vi "V1.0 Convert.vi"(11 "Old":T17 {"AllCaliperEntries"."CaliperType" items=["Distance", "Mid Point", "Perpendicular Projection", "Lines Intersection", "Angle from Horizontal", "Angle from Vertical", "Angle Defined by 3 Points", "Angle Defined by 4 Points", "Bissecting Line", "Mid Line", "Center of Mass", "Area", "Line Fit", "Circle Fit", "Ellipse Fit"]; "CoordinatteEntry Output"."AnalysisSetting"."OriginPointInfo"."Mode" items=["Horizontal Motion", "Vertical Motion", "Horizontal and Vertical Motion", "Horizontal. Vertical and Angular Motion"]; "CoordinatteEntry Output"."AnalysisSetting"."ROI"."Contours"."Type" items=["No Selection", "Point", "Line", "Rectangle", "Oval", "Polygon", "Freehand Region", "Annulus", "Unused2", "Unused3", "Broken Line", "Freehand Line", "Rotated Rectangle"]; "AllCaliperEntries"."CaliperType" items=["Distance", "Mid Point", "Perpendicular Projection", "Lines Intersection", "Angle from Horizontal", "Angle from Vertical", "Angle Defined by 3 Points", "Angle Defined by 4 Points", "Bissecting Line", "Mid Line", "Center of Mass", "Area", "Line Fit", "Circle Fit", "Ellipse Fit"]}) -> (3 "NewOut":T16 {"AllCaliperEntries"."CaliperType" items=["Distance", "Mid Point", "Perpendicular Projection", "Lines Intersection", "Angle from Horizontal", "Angle from Vertical", "Angle Defined by 3 Points", "Angle Defined by 4 Points", "Bissecting Line", "Mid Line", "Center of Mass", "Area", "Line Fit", "Circle Fit", "Ellipse Fit"]; "CoordinatteEntry Output"."CaliperSetting"."CaliperEntry"."CaliperType" items=["Distance", "Mid Point", "Perpendicular Projection", "Lines Intersection", "Angle from Horizontal", "Angle from Vertical", "Angle Defined by 3 Points", "Angle Defined by 4 Points", "Bissecting Line", "Mid Line", "Center of Mass", "Area", "Line Fit", "Circle Fit", "Ellipse Fit"]; "CoordinatteEntry Output"."OriginPointInfo"."Mode" items=["Horizontal Motion", "Vertical Motion", "Horizontal and Vertical Motion", "Horizontal. Vertical and Angular Motion"]; "CoordinatteEntry Output"."AnalysisSetting"."ROI"."Contours"."Type" items=["No Selection", "Point", "Line", "Rectangle", "Oval", "Polygon", "Freehand Region", "Annulus", "Unused2", "Unused3", "Broken Line", "Freehand Line", "Rotated Rectangle"]; "AllCaliperEntries"."CaliperType" items=["Distance", "Mid Point", "Perpendicular Projection", "Lines Intersection", "Angle from Horizontal", "Angle from Vertical", "Angle Defined by 3 Points", "Angle Defined by 4 Points", "Bissecting Line", "Mid Line", "Center of Mass", "Area", "Line Fit", "Circle Fit", "Ellipse Fit"]})   [LabVIEW 2019]
uses:
  Process/Controls/Process_Setting.ctl
  Coordinate/Control/CoordinateAnalysisSetting.ctl
  Caliper/Controls/CaliperType.ctl
  Caliper/Controls/SelectionListEntryPointType.ctl
  Caliper/Controls/SelectionListEntry.ctl
  Caliper/Controls/CaliperResult.ctl
  Caliper/Controls/CaliperDataEntry.ctl
  Coordinate/Control/CoordinateCaliperSetting.ctl
  Coordinate/Control/CoordinatteEntry.ctl
  Controls/ParameterData.ctl
  Analysis/Controls/Analysis_Setting.ctl
  Controls/Vision_DataEntry.ctl
  Analysis/Controls/V_Analysis_Type.ctl
  Ctrl/VisionProcessName.ctl
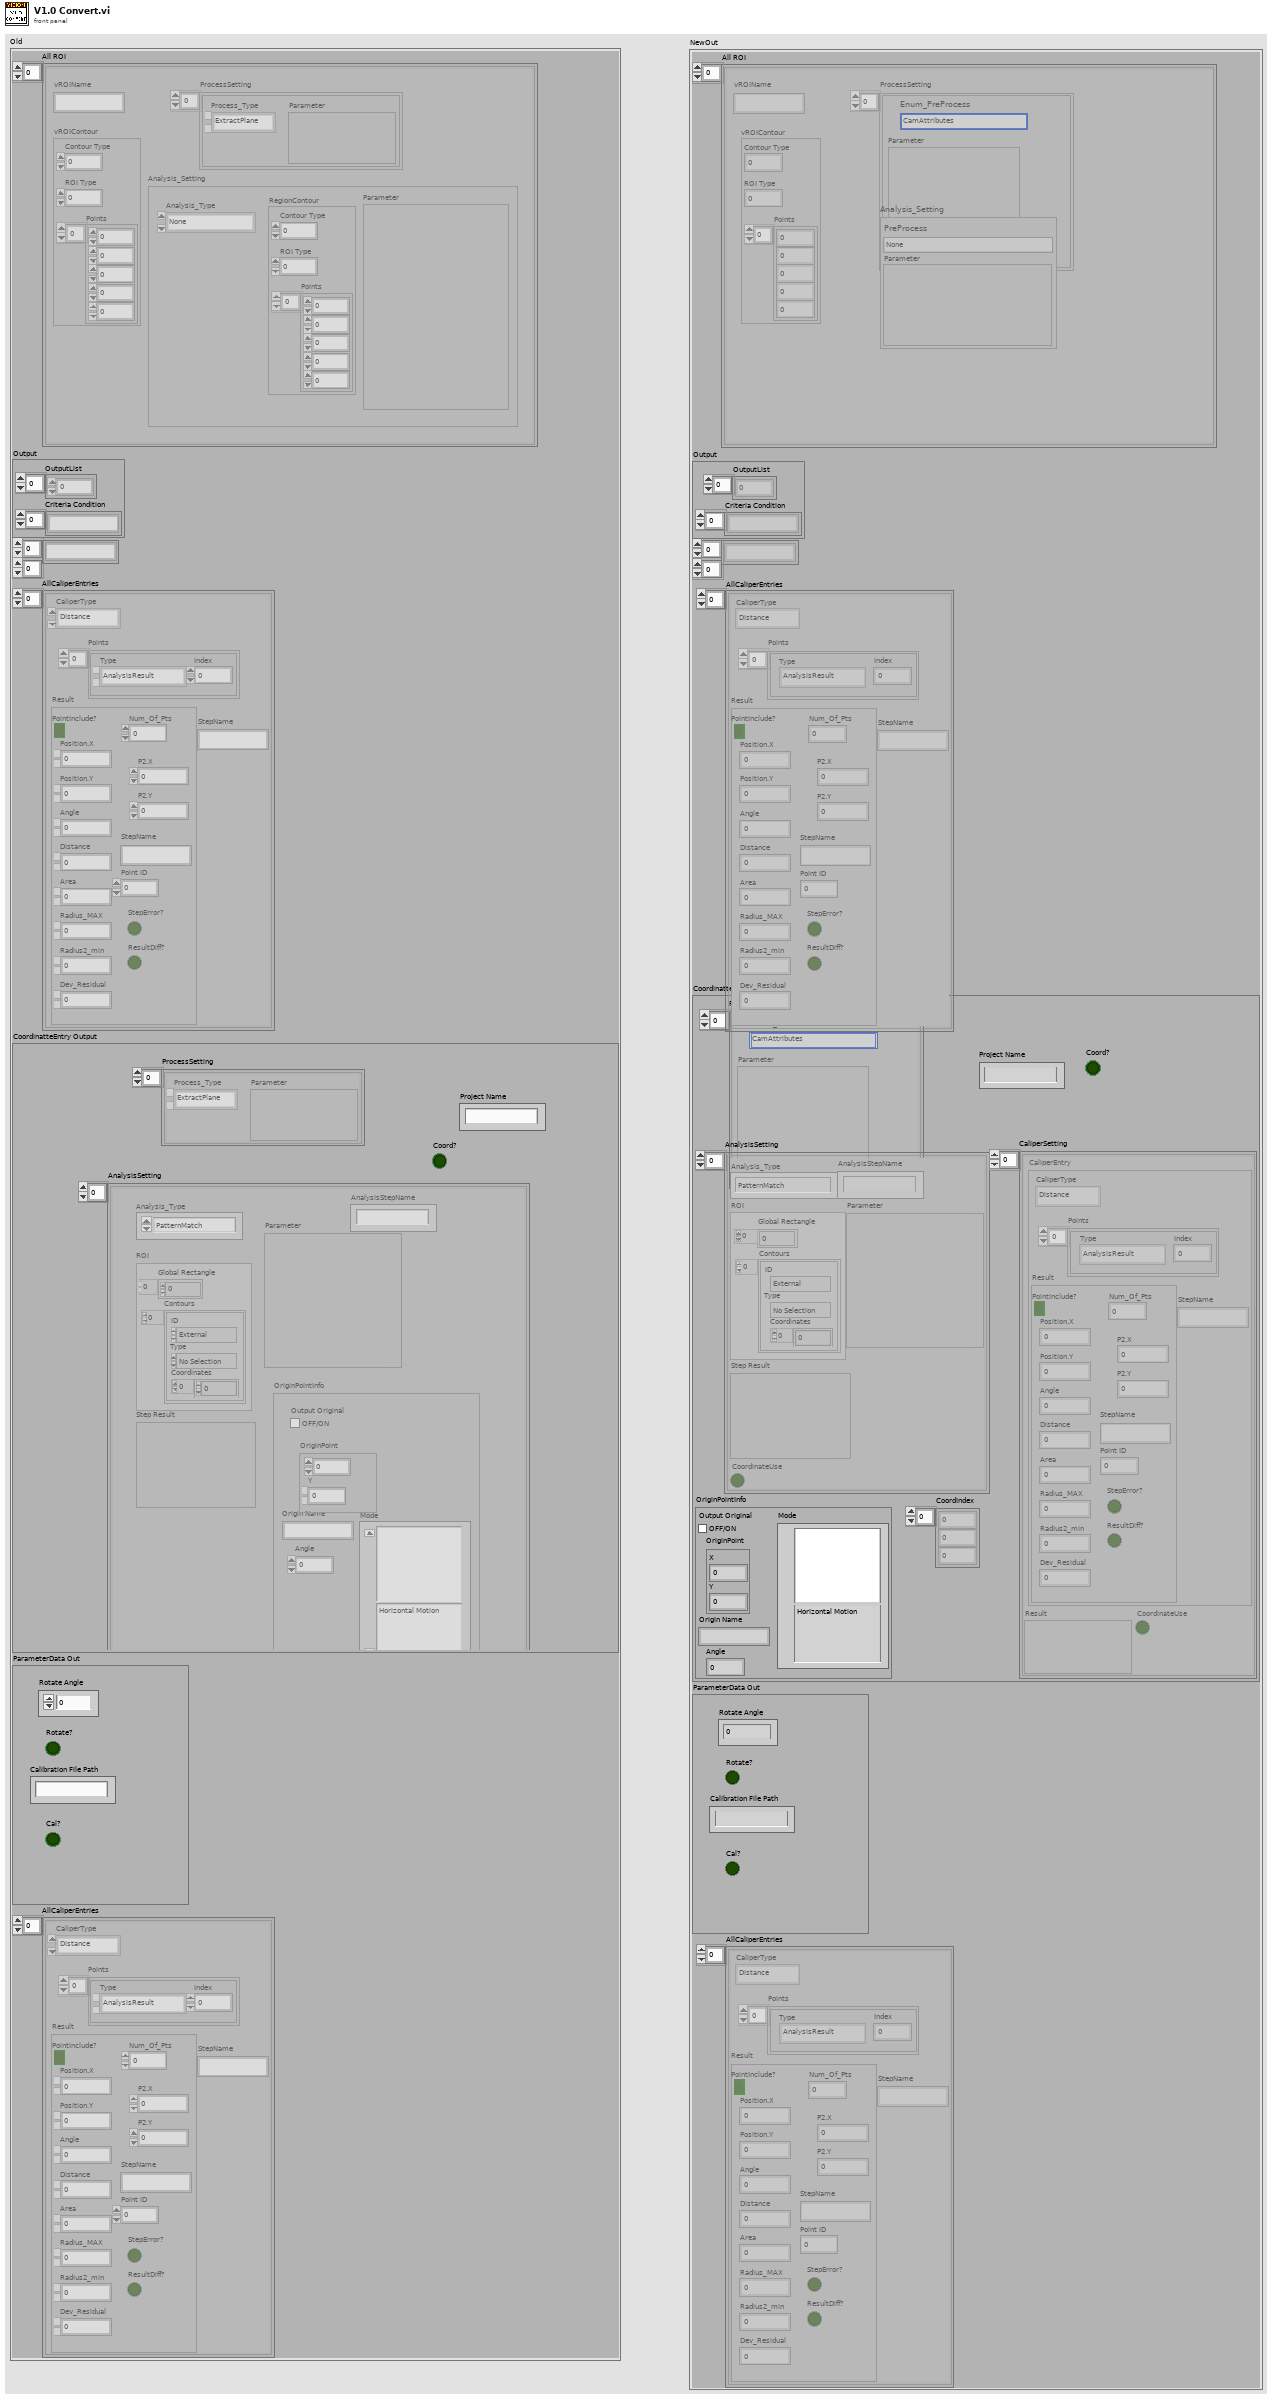
[diagram p1: front panel]
types:
  T1 = typedef "Vision_DataEntry.ctl" = cluster{"vROIName":string, "vROIContour":cluster{"Contour Type":u32, "ROI Type":u32, "Points":i32[]}, "ProcessSetting":T2[], "Analysis_Setting":T4}
  T2 = typedef "Process_Setting.ctl" = cluster{"Enum_PreProcess":T3, "Parameter":string}
  T3 = typedef "VisionProcessName.ctl" = enum16{"*CamParameter*", "CamAttributes", "*Preprocess*", "CG_Brightness", "C_Plane Extraction", "C_Threshold", "G_Lookup Table", "G_Threshold"}
  T4 = typedef "Analysis_Setting.ctl" = cluster{"PreProcess":T5, "Parameter":string}
  T5 = typedef "V_Analysis_Type.ctl" = enum16{"None", "C_Color Pattern Matching", "G_PatternMatching", "G_ShapeDectect", "G_GeometricMatch", "B_Area Check"}
  T6 = typedef "CaliperDataEntry.ctl" = cluster{"CaliperType":T7, "Points":T8[], "Result":T10, "StepName":string}
  T7 = typedef "CaliperType.ctl" = u32
  T8 = typedef "SelectionListEntry.ctl" = cluster{"Type":T9, "Index":i32}
  T9 = typedef "SelectionListEntryPointType.ctl" = enum16{"AnalysisResult", "CaliperResult"}
  T10 = typedef "CaliperResult.ctl" = cluster{"PointInclude?":bool, "Num_Of_Pts":u8, "Position.X":dbl, "Position.Y":dbl, "Angle":dbl, "Distance":dbl, "Area":dbl, "Radius_MAX":dbl, "Radius2_min":dbl, "Dev_Residual":dbl, "P2.X":dbl, "P2.Y":dbl, "StepName":string, "Point ID":u8, "StepError?":bool, "ResultDiff?":bool}
  T11 = typedef "CoordinatteEntry.ctl" = cluster{"ProcessSetting":T2[], "Project Name":string, "AnalysisSetting":T12[], "Coord?":bool, "OriginPointInfo":cluster{"Output Original":bool, "Origin Name":string, "Angle":dbl, "Mode":u16, "OriginPoint":cluster{"X":dbl, "Y":dbl}}, "CaliperSetting":T14[], "CoordIndex":i32[]}
  T12 = typedef "CoordinateAnalysisSetting.ctl" = cluster{"Analysis_Type":enum16{"PatternMatch", "Straight Edge"}, "ROI ":T13, "Parameter":variant, "Step Result":variant, "AnalysisStepName":string, "CoordinateUse":bool}
  T13 = typedef "ROI Descriptor" = cluster{"Global Rectangle":i32[], "Contours":cluster{"ID":enum32{"External", "Internal"}, "Type":u32, "Coordinates":i32[]}[]}
  T14 = typedef "CoordinateCaliperSetting.ctl" = cluster{"Result":variant, "CoordinateUse":bool, "CaliperEntry":T6}
  T15 = typedef "ParameterData.ctl" = cluster{"Rotate Angle":dbl, "Rotate?":bool, "Calibration File Path":string, "Cal?":bool}
  T16 = cluster{"All ROI":T1[], "Output":cluster{"OutputList":u16[], "Criteria Condition":string[]}, string[][], "AllCaliperEntries":T6[], "CoordinatteEntry Output":T11, "ParameterData Out":T15, "AllCaliperEntries":T6[]}
  T17 = cluster{"All ROI":cluster{"vROIName":string, "vROIContour":cluster{"Contour Type":u32, "ROI Type":u32, "Points":i32[]}, "ProcessSetting":cluster{"Process_Type":enum16{"None", "ExtractPlane", "BinaryMono", "Operators", "GrayMorphology", "Filters", "Lookup Table", "Particle Filter", "Mask"}, "Parameter":variant}[], "Analysis_Setting":cluster{"Analysis_Type":enum16{"None", "PatternMatch", "Edge Detection", "Barcode 1D", "Barcode 2D", "Clamp", "Clamp MAX", "Particle", "Histogram", "Straight Edge", "Circle", "Shape Dectect", "OCR"}, "RegionContour":cluster{"Contour Type":u32, "ROI Type":u32, "Points":i32[]}, "Parameter":variant}}[], "Output":cluster{"OutputList":u16[], "Criteria Condition":string[]}, string[][], "AllCaliperEntries":cluster{"CaliperType":u32, "Points":cluster{"Type":enum16{"AnalysisResult", "CaliperResult"}, "Index":i32}[], "Result":cluster{"PointInclude?":bool, "Num_Of_Pts":u8, "Position.X":dbl, "Position.Y":dbl, "Angle":dbl, "Distance":dbl, "Area":dbl, "Radius_MAX":dbl, "Radius2_min":dbl, "Dev_Residual":dbl, "P2.X":dbl, "P2.Y":dbl, "StepName":string, "Point ID":u8, "StepError?":bool, "ResultDiff?":bool}, "StepName":string}[], "CoordinatteEntry Output":cluster{"ProcessSetting":cluster{"Process_Type":enum16{"None", "ExtractPlane", "BinaryMono", "Operators", "GrayMorphology", "Filters", "Lookup Table", "Particle Filter", "Mask"}, "Parameter":variant}[], "Project Name":string, "AnalysisSetting":cluster{"Analysis_Type":enum16{"PatternMatch", "Straight Edge"}, "ROI ":T13, "Parameter":variant, "Step Result":variant, "OriginPointInfo":cluster{"Output Original":bool, "Origin Name":string, "Angle":dbl, "Mode":u16, "OriginPoint":cluster{"X":dbl, "Y":dbl}}, "AnalysisStepName":string}[], "Coord?":bool}, "ParameterData Out":cluster{"Rotate Angle":dbl, "Rotate?":bool, "Calibration File Path":string, "Cal?":bool}, "AllCaliperEntries":cluster{"CaliperType":u32, "Points":cluster{"Type":enum16{"AnalysisResult", "CaliperResult"}, "Index":i32}[], "Result":cluster{"PointInclude?":bool, "Num_Of_Pts":u8, "Position.X":dbl, "Position.Y":dbl, "Angle":dbl, "Distance":dbl, "Area":dbl, "Radius_MAX":dbl, "Radius2_min":dbl, "Dev_Residual":dbl, "P2.X":dbl, "P2.Y":dbl, "StepName":string, "Point ID":u8, "StepError?":bool, "ResultDiff?":bool}, "StepName":string}[]}
  T18 = cluster{"Output Original":bool, "Origin Name":string, "Angle":dbl, "Mode":u16, "OriginPoint":cluster{"X":dbl, "Y":dbl}}
  T19 = cluster{"vROIName":string, "vROIContour":cluster{"Contour Type":u32, "ROI Type":u32, "Points":i32[]}, "ProcessSetting":cluster{"Process_Type":enum16{"None", "ExtractPlane", "BinaryMono", "Operators", "GrayMorphology", "Filters", "Lookup Table", "Particle Filter", "Mask"}, "Parameter":variant}[], "Analysis_Setting":cluster{"Analysis_Type":enum16{"None", "PatternMatch", "Edge Detection", "Barcode 1D", "Barcode 2D", "Clamp", "Clamp MAX", "Particle", "Histogram", "Straight Edge", "Circle", "Shape Dectect", "OCR"}, "RegionContour":cluster{"Contour Type":u32, "ROI Type":u32, "Points":i32[]}, "Parameter":variant}}[]
  T20 = cluster{"OutputList":u16[], "Criteria Condition":string[]}
  T21 = cluster{"CaliperType":u32, "Points":cluster{"Type":enum16{"AnalysisResult", "CaliperResult"}, "Index":i32}[], "Result":cluster{"PointInclude?":bool, "Num_Of_Pts":u8, "Position.X":dbl, "Position.Y":dbl, "Angle":dbl, "Distance":dbl, "Area":dbl, "Radius_MAX":dbl, "Radius2_min":dbl, "Dev_Residual":dbl, "P2.X":dbl, "P2.Y":dbl, "StepName":string, "Point ID":u8, "StepError?":bool, "ResultDiff?":bool}, "StepName":string}[]
  T22 = cluster{"Process_Type":enum16{"None", "ExtractPlane", "BinaryMono", "Operators", "GrayMorphology", "Filters", "Lookup Table", "Particle Filter", "Mask"}, "Parameter":variant}[]
  T23 = cluster{"Analysis_Type":enum16{"PatternMatch", "Straight Edge"}, "ROI ":T13, "Parameter":variant, "Step Result":variant, "OriginPointInfo":cluster{"Output Original":bool, "Origin Name":string, "Angle":dbl, "Mode":u16, "OriginPoint":cluster{"X":dbl, "Y":dbl}}, "AnalysisStepName":string}[]
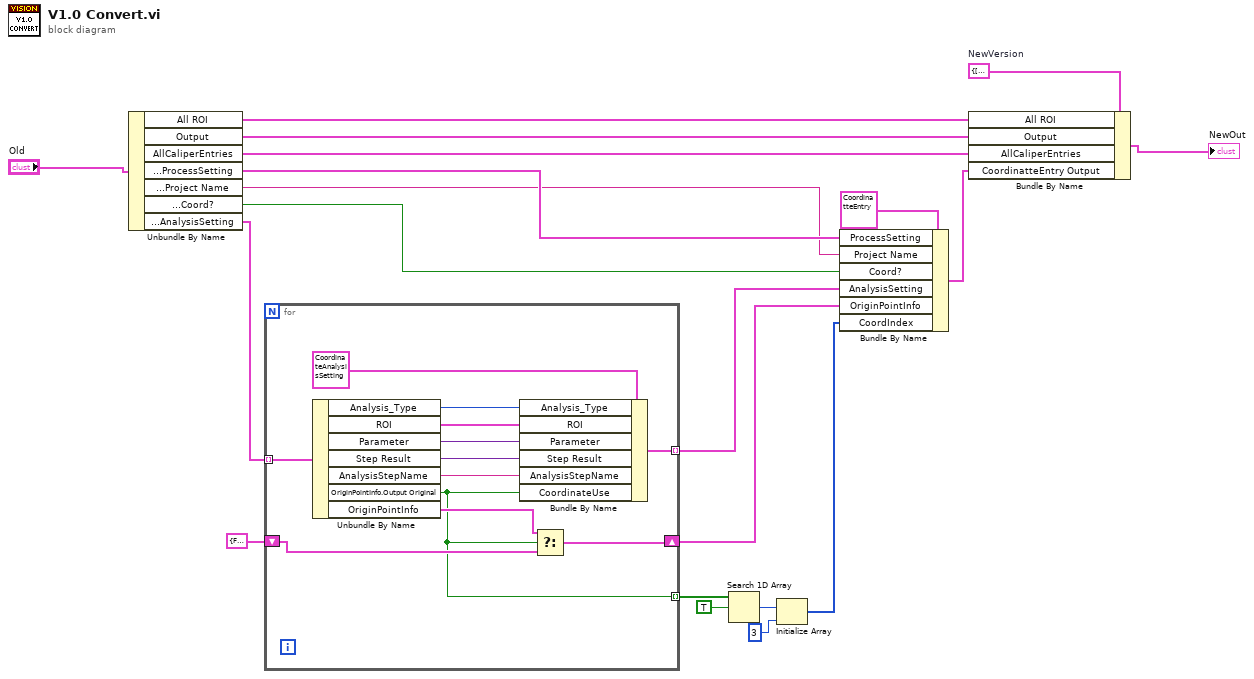
[diagram p0: block diagram]
diagram:
  w3 = T16 {"All ROI"=[], "Output"={"OutputList"=[], "Criteria Condition"=[]}, [], "AllCaliperEntries"=[], "CoordinatteEntry Output"={"ProcessSetting"=[], "Project Name"="", "AnalysisSetting"=[], "Coord?"=FALSE, "OriginPointInfo"={"Output Original"=FALSE, "Origin Name"="", "Angle"=0.0, "Mode"=0, "OriginPoint"={"X"=0.0, "Y"=0.0}}, "CaliperSetting"=[], "CoordIndex"=[]}, "ParameterData Out"={"Rotate Angle"=0.0, "Rotate?"=FALSE, "Calibration File Path"="", "Cal?"=FALSE}, "AllCaliperEntries"=[]}  # NewVersion
  n1 = Unbundle By Name("Old") -> ("All ROI"=w20:T19, "Output"=w19:T20, "AllCaliperEntries"=w18:T21, "CoordinatteEntry Output.ProcessSetting"=w16:T22, "CoordinatteEntry Output.Project Name"=w15:string, "CoordinatteEntry Output.Coord?"=w13:bool, "CoordinatteEntry Output.AnalysisSetting"=w12:T23)
  n2 = for {
    tunnel: w12 -> [w32] mode=indexing
    tunnel: [w25] -> w11 mode=indexing
    shift-right: [w23] -> w9
    shift-left: T18 {"Output Original"=FALSE, "Origin Name"="", "Angle"=0.0, "Mode"=0, "OriginPoint"={"X"=0.0, "Y"=0.0}} ("OriginPointInfo") -> [w22]
    tunnel: [w21] -> w8 mode=indexing
    n3 = Unbundle By Name(w32) -> ("Analysis_Type"=w30:enum16{"PatternMatch", "Straight Edge"}, "ROI"=w29:T13, "Parameter"=w28:variant, "Step Result"=w27:variant, "AnalysisStepName"=w26:string, "OriginPointInfo.Output Original"=w21:bool, "OriginPointInfo"=w24:T18)
    n4 = Bundle By Name(cluster=T12 {"Analysis_Type"=enum."PatternMatch", "ROI "={"Global Rectangle"=[], "Contours"=[]}, "Parameter"=variant, "Step Result"=variant, "AnalysisStepName"="", "CoordinateUse"=FALSE} ("CoordinateAnalysisSetting"), "Analysis_Type"=w30, "ROI"=w29, "Parameter"=w28, "Step Result"=w27, "AnalysisStepName"=w26, "CoordinateUse"=w21) -> (w25:T12)
    n5 = Select(t=w24, s=w21, f=w22) -> (s? t:f=w23:T18)
  }
  n6 = Search 1D Array(1D array=w8, element=TRUE) -> (index of element=w6:i32)  [unwired: 1 in]
  n7 = Initialize Array(w6, 3 ("dimension size")) -> (w4:i32[])
  n8 = Bundle By Name(cluster=T11 {"ProcessSetting"=[], "Project Name"="", "AnalysisSetting"=[], "Coord?"=FALSE, "OriginPointInfo"={"Output Original"=FALSE, "Origin Name"="", "Angle"=0.0, "Mode"=0, "OriginPoint"={"X"=0.0, "Y"=0.0}}, "CaliperSetting"=[], "CoordIndex"=[]} ("CoordinatteEntry Output"), "ProcessSetting"=w16, "Project Name"=w15, "Coord?"=w13, "AnalysisSetting"=w11, "OriginPointInfo"=w9, "CoordIndex"=w4) -> (w14:T11)
  n9 = Bundle By Name(cluster=w3, "All ROI"=w20, "Output"=w19, "AllCaliperEntries"=w18, "CoordinatteEntry Output"=w14) -> (→"NewOut":T16)
